vi "CRYGet Language.vi"   [LabVIEW 2013]
uses:
  CRYMainGlobal.vi
  Kernel32.DLL
types:
  T1 = enum32{"English", "Chinese", "Korean", "Japanese", "Russian", "Chinese traditional"}
  T2 = cluster{"Section":string, "Items":cluster{"Key":string, "Value":string}[]}[]
  T3 = cluster{"Section":string, "Items":cluster{"Key":string, "Value":string}[]}
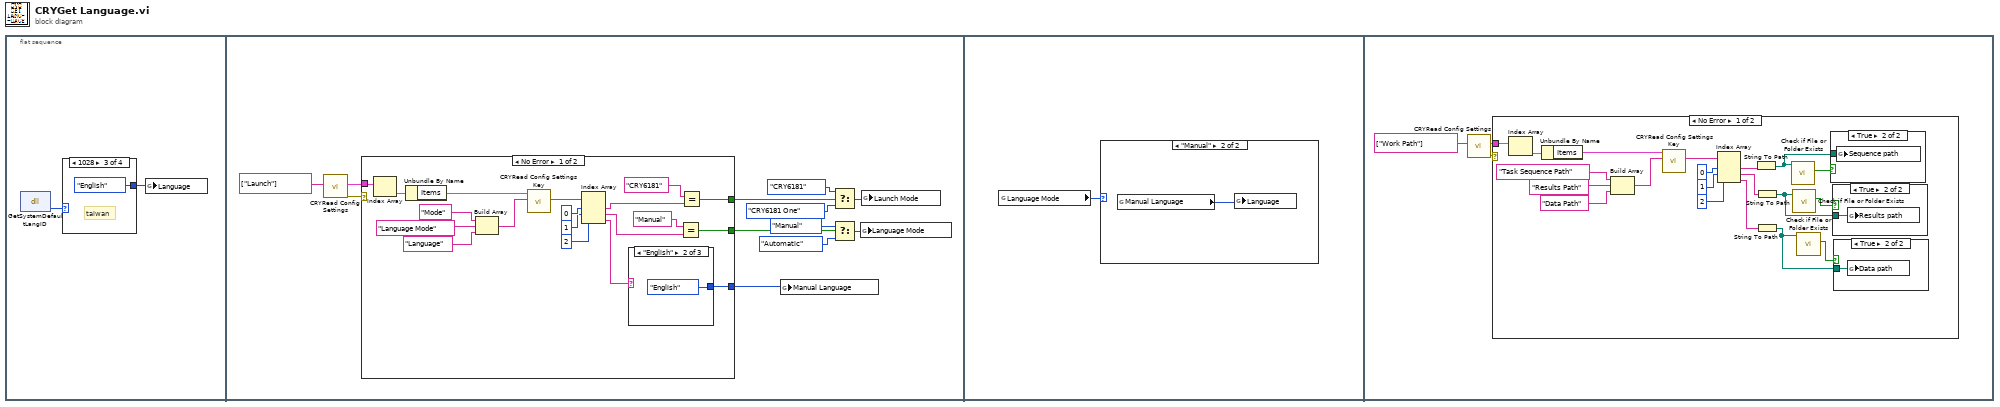
[diagram p0: block diagram]
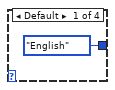
[diagram p2: hidden frame]
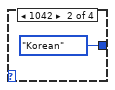
[diagram p3: hidden frame]
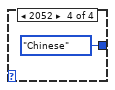
[diagram p4: hidden frame]
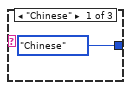
[diagram p5: hidden frame]
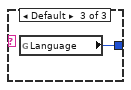
[diagram p6: hidden frame]
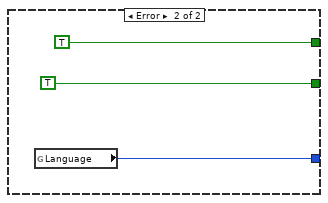
[diagram p7: hidden frame]
diagram:
  n1 = flat-sequence {
    frame #0 {
      n2 = dll-call lib="kernel32.dll" fn="GetSystemDefaultLangID"() -> ("return type"=w2:u16)  [unwired: 3 in, 2 out]
      n3 = case shown="1028" w2 {
        tunnel: [T1."English" ("Language") T1."Korean" ("Language") T1."English" ("Language") T1."Chinese" ("Language")] -> w1
        frame Default {
        }
        frame 1042 {
        }
        frame 1028 {
          # "taiwan"
        }
        frame 2052 {
        }
      }
      n4 = global write "CRYMainGlobal.vi" "Language"(w1) -> ()
    }
    frame #1 {
      n5 = call "CRYRead Config Settings.vi"("Section"=string[] ["Launch"]) -> ("error out"=w11:errorcluster, "Configuration Data"=w9:T2)  [unwired: 9 in]
      n6 = case shown="No Error" w11 {
        tunnel: w9 -> [w37 _]
        tunnel: [w34 TRUE] -> w10
        tunnel: [w29 TRUE] -> w15
        tunnel: [w28 w41] -> w7
        frame No Error {
          n7 = Index Array(array=w37) -> (element=w36:T3)  [unwired: 1 in]
          n8 = Unbundle By Name(w36) -> ("Items"=w23:cluster{"Key":string, "Value":string}[])
          n9 = Build Array("Mode" ("Section"), "Language Mode" ("Section"), "Language" ("Section")) -> (w24:string[])
          n10 = call "CRYRead Config Settings Key.vi"("Key Names"=w24, "Items"=w23) -> ("Values"=w22:string[])  [unwired: 9 in]
          n11 = Index Array(array=w22, index #1=0 ("index"), index #2=1 ("index"), index #3=2 ("index")) -> (element #1=w21:string, element #2=w20:string, element #3=w19:string)
          n12 = case shown="\"English\"" w19 {
            tunnel: [enum32{"English", "Chinese"}."Chinese" ("Manual Language") enum32{"English", "Chinese"}."English" ("Manual Language") w40] -> w28
            frame "Chinese" {
            }
            frame "English" {
            }
            frame Default {
              n13 = global read "CRYMainGlobal.vi" "Language"() -> (w40:T1)
            }
          }
          n14 = Equal?(x="Manual", y=w20) -> (x = y?=w29:bool)
          n15 = Equal?(x="CRY6181" ("Section"), y=w21) -> (x = y?=w34:bool)
        }
        frame Error {
          n16 = global read "CRYMainGlobal.vi" "Language"() -> (w41:T1)
        }
      }
      n17 = global write "CRYMainGlobal.vi" "Manual Language"(w7) -> ()
      n18 = Select(t=enum32{"CRY6181", "CRY6181 One"}."CRY6181" ("Launch Mode"), s=w10, f=enum32{"CRY6181", "CRY6181 One"}."CRY6181 One" ("Launch Mode")) -> (s? t:f=w14:enum32{"CRY6181", "CRY6181 One"})
      n19 = Select(t=enum32{"Automatic", "Manual"}."Manual" ("Language Mode"), s=w15, f=enum32{"Automatic", "Manual"}."Automatic") -> (s? t:f=w17:enum32{"Automatic", "Manual"})
      n20 = global write "CRYMainGlobal.vi" "Language Mode"(w17) -> ()
      n21 = global write "CRYMainGlobal.vi" "Launch Mode"(w14) -> ()
    }
    frame #2 {
      n22 = global read "CRYMainGlobal.vi" "Language Mode"() -> (w44:enum32{"Automatic", "Manual"})
      n23 = case shown="\"Manual\"" w44 {
        frame "Automatic", Default {
        }
        frame "Manual" {
          n24 = global read "CRYMainGlobal.vi" "Manual Language"() -> (w45:enum32{"English", "Chinese"})
          n25 = global write "CRYMainGlobal.vi" "Language"(w45) -> ()
        }
      }
    }
    frame #3 {
      n26 = call "CRYRead Config Settings.vi"("Section"=string[] ["Work Path"]) -> ("error out"=w46:errorcluster, "Configuration Data"=w47:T2)  [unwired: 9 in]
      n27 = case shown="No Error" w46 {
        tunnel: w47 -> [w68 _]
        frame No Error {
          n28 = Index Array(array=w68) -> (element=w67:T3)  [unwired: 1 in]
          n29 = Unbundle By Name(w67) -> ("Items"=w59:cluster{"Key":string, "Value":string}[])
          n30 = Build Array("Task Sequence Path" ("Section"), "Results Path" ("Section"), "Data Path" ("Section")) -> (w60:string[])
          n31 = call "CRYRead Config Settings Key.vi"("Key Names"=w60, "Items"=w59) -> ("Values"=w58:string[])  [unwired: 9 in]
          n32 = Index Array(array=w58, index #1=0 ("index"), index #2=1 ("index"), index #3=2 ("index")) -> (element #1=w57:string, element #2=w56:string, element #3=w55:string)
          n33 = String To Path(string=w57) -> (path=w53:path)
          n34 = String To Path(string=w56) -> (path=w52:path)
          n35 = String To Path(string=w55) -> (path=w50:path)
          n36 = call <vilib>:"Check if File or Folder Exists.vi"("path"=w53) -> ("file or folder exists?"=w54:bool)  [unwired: 8 in, 2 out]
          n37 = call <vilib>:"Check if File or Folder Exists.vi"("path"=w52) -> ("file or folder exists?"=w51:bool)  [unwired: 8 in, 2 out]
          n38 = call <vilib>:"Check if File or Folder Exists.vi"("path"=w50) -> ("file or folder exists?"=w49:bool)  [unwired: 8 in, 2 out]
          n39 = case shown="True" w54 {
            tunnel: w53 -> [_ w71]
            frame False {
            }
            frame True {
              n40 = global write "CRYMainGlobal.vi" "Sequence path"(w71) -> ()
            }
          }
          n41 = case shown="True" w51 {
            tunnel: w52 -> [_ w70]
            frame False {
            }
            frame True {
              n42 = global write "CRYMainGlobal.vi" "Results path"(w70) -> ()
            }
          }
          n43 = case shown="True" w49 {
            tunnel: w50 -> [_ w69]
            frame False {
            }
            frame True {
              n44 = global write "CRYMainGlobal.vi" "Data path"(w69) -> ()
            }
          }
        }
        frame Error {
        }
      }
    }
  }
